vi "Configure Flow Rate.vi"(0 "VISA resource name":refnum<visa-resource-name>="COM1", 5 "Address (00)":i32 format="%0#2.0f", 7 "Flow Rate (100)":dbl=100.0, 9 "Units (0: microliters per minute)":u16(ring) items=["microliters per minute (ul/min.)", "microliters per hour (ul/hr.)", "milliliters per minute (ml/min.)", "milliliters per hour (ml/hr.)", "picoliters per minute (pl/min.)", "picoliters per hour (pl/hr.)", "nanoliters per minute (nl/min.)", "nanoliters per hour (nl/hr.)"], 11 "error in (no error)":errorcluster, 12 "Pump direction":enum16{"Infuse", "Withdraw"}(ring)) -> (4 "VISA resource name out":refnum<visa-resource-name>, 15 "error out":errorcluster)   [LabVIEW 2015]
doc: "This VI will set the flow rate of the pump. \nModified from original which is Copyright 2005, National Instruments Corporation"
panel:
  out "Command":string
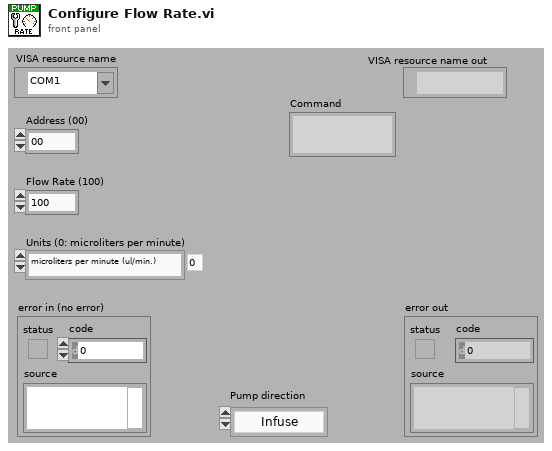
[diagram p1: front panel]
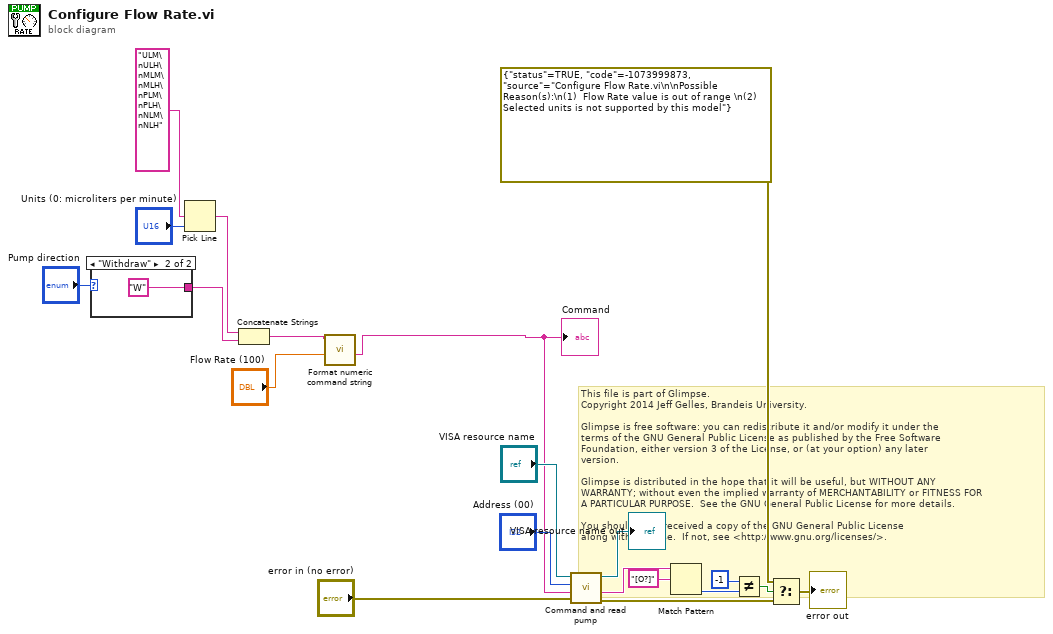
[diagram p0: block diagram]
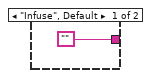
[diagram p2: hidden frame]
diagram:
  # "This file is part of Glimpse. \nCopyright 2014 Jeff Gelles, Brandeis University.    \n\nGlimpse is free software: you can redistribute it and/or modify it under the \nterms of the GNU General Public License as published by the Free Software \nFoundation, either version 3 of the License, or (at your option) any later \nversion.\n\nGlimpse is distributed in the hope that it will be useful, but WITHOUT ANY \nWARRANTY; without even the implied warranty of MERCHANTABILITY or FITNESS FOR \nA PARTICULAR PURPOSE.  See the GNU General Public License for more details.\n\nYou should have received a copy of the GNU General Public License\nalong with Glimpse.  If not, see <http://www.gnu.org/licenses/>."
  n1 = case shown="\"Withdraw\"" "Pump direction" {
    tunnel: ["" "W"] -> w10
    frame "Infuse", Default {
    }
    frame "Withdraw" {
    }
  }
  n2 = Pick Line(multi-line string="ULM\nULH\nMLM\nMLH\nPLM\nPLH\nNLM\nNLH", line index="Units (0: microliters per minute)") -> (output string=w11:string)  [unwired: 1 out]
  n3 = Concatenate Strings(w11, w10) -> (w4:string)
  n4 = call "Format numeric command string.vi"("Number"="Flow Rate (100)", "Command"=w4) -> ("String"=w1:string)  [unwired: 5 out]
  "Command" <- w1
  n5 = call "Command and read pump.vi"("error in (no error)"="error in (no error)", "command"=w1, "Address (00)"="Address (00)", "VISA resource name"="VISA resource name") -> ("error out"=w7:errorcluster, "Output String"=w5:string, "VISA resource name out"=→"VISA resource name out":refnum<visa-resource-name>)  [unwired: 5 out]
  n6 = Match Pattern(string=w5, regular expression="[O?]") -> (offset past match=w18:i32)  [unwired: 4 out]
  n7 = Not Equal?(x=-1, y=w18) -> (x != y?=w16:bool)
  n8 = Select(t=errorcluster {"status"=TRUE, "code"=-1073999873, "source"="Configure Flow Rate.vi\n\nPossible Reason(s):\n(1)  Flow Rate value is out of range \n(2)  Selected units is not supported by this model"}, s=w16, f=w7) -> (s? t:f=→"error out":errorcluster)
